vi "set channel info.vi"(8 "error in (no error)":errorcluster, 9 "channel info":T1, 10 "id":string, 11 "DSFConfiguration in":refnum<class "DSFConfiguration.lvclass">) -> (0 "error out":errorcluster, 3 "DSFConfiguration out":refnum<class "DSFConfiguration.lvclass">)   [LabVIEW 2017, in "DSFConfiguration.lvclass"]
uses:
  DSFConfiguration.lvclass
  Controls/dsf channel.ctl
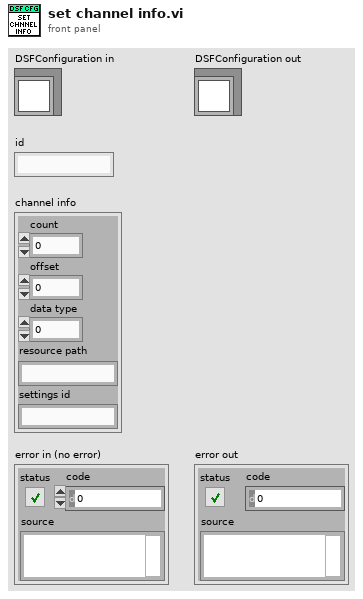
[diagram p1: front panel]
types:
  T1 = typedef "dsf channel.ctl" = cluster{"count":i32, "offset":i32, "data type":i32, "resource path":string, "settings id":string}
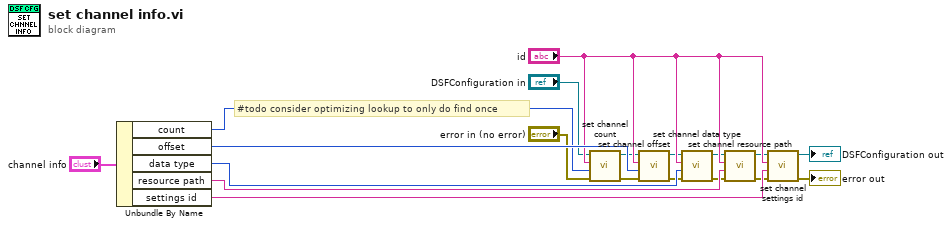
[diagram p0: block diagram]
diagram:
  # "#todo consider optimizing lookup to only do find once"
  n1 = Unbundle By Name("channel info") -> ("count"=w3:i32, "offset"=w16:i32, "data type"=w17:i32, "resource path"=w18:string, "settings id"=w19:string)
  n2 = call "set channel count.vi"("error in (no error)"="error in (no error)", "count"=w3, "id"="id", "DSFConfiguration in"="DSFConfiguration in") -> ("error out"=w6:errorcluster, "DSFConfiguration out"=w5:refnum<class "DSFConfiguration.lvclass">)  [unwired: 6 in]
  n3 = call "set channel offset.vi"("error in (no error)"=w6, "offset"=w16, "id"="id", "DSFConfiguration in"=w5) -> ("error out"=w8:errorcluster, "DSFConfiguration out"=w7:refnum<class "DSFConfiguration.lvclass">)  [unwired: 6 in]
  n4 = call "set channel data type.vi"("error in (no error)"=w8, "data type"=w17, "id"="id", "DSFConfiguration in"=w7) -> ("error out"=w10:errorcluster, "DSFConfiguration out"=w9:refnum<class "DSFConfiguration.lvclass">)  [unwired: 6 in]
  n5 = call "set channel resource path.vi"("error in (no error)"=w10, "vs channel path"=w18, "id"="id", "DSFConfiguration in"=w9) -> ("error out"=w12:errorcluster, "DSFConfiguration out"=w11:refnum<class "DSFConfiguration.lvclass">)  [unwired: 6 in]
  n6 = call "set channel settings id.vi"("error in (no error)"=w12, "settings id"=w19, "id"="id", "DSFConfiguration in"=w11) -> ("error out"=→"error out":errorcluster, "DSFConfiguration out"=→"DSFConfiguration out":refnum<class "DSFConfiguration.lvclass">)  [unwired: 6 in]
